vi "Write Action Type and Number.vi"(8 "error in (no error)":errorcluster, 9 "Action Number":i32[](array[numeric]), 10 "Action Type":T1, 11 "Project Action in":refnum<class "Project Action.lvclass">) -> (0 "error out":errorcluster, 3 "Project Action out":refnum<class "Project Action.lvclass">)   [LabVIEW 2019, in "ProjectBuilder.lvlib" / "Project Action.lvclass"]
doc: "Write 'Action Type' and 'Action Number' to the private data."
uses:
  Project Action.lvclass
  Ctl/Ctl_Build Steps.ctl
  ProjectBuilder.lvlib
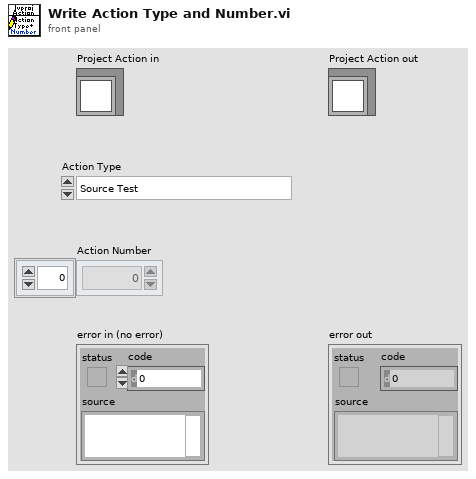
[diagram p1: front panel]
types:
  T1 = typedef "ProjectBuilder.lvlib/Ctl_Build Steps.ctl" = enum16{"Source Test", "Build", "Post-Build Test", "Deploy", "Report"}
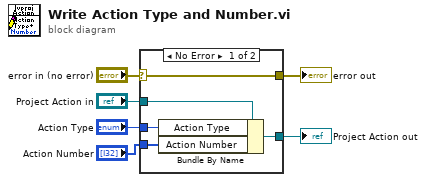
[diagram p0: block diagram]
diagram:
  n1 = case shown="No Error" "error in (no error)" {
    selector: "error in (no error)" -> [w11 w12]
    tunnel: [w11 w12] -> w5
    tunnel: [w9 w13] -> w3
    tunnel: "Project Action in" -> [w10 w13]
    tunnel: "Action Type" -> [w8 _]
    tunnel: "Action Number" -> [w7 _]
    frame No Error {
      n2 = Bundle By Name(cluster=w10, "Action Type"=w8, "Action Number"=w7) -> (w9:refnum<class "Project Action.lvclass">)
    }
    frame Error {
    }
  }
  "error out" <- w5
  "Project Action out" <- w3
